vi "READ_SCOPETRACESENErgz analysis.vi"() -> ()   [LabVIEW 2011]
panel:
  out "results":dbl[][](array[numeric])
  out "Array":dbl[](array[numeric])
  in  "Export folder":bool
  in  "Export file":bool
  in  "Files":i32[](listbox)=[7]
  out "filenames":string[](array[string])=["TREX PXI slow_026.dat", "TREX PXI slow_027.dat", "TREX PXI slow_028.dat", "TREX PXI slow_029.dat", "TREX PXI slow_030.dat", "TREX PXI slow_031.dat", "TREX PXI slow_032.dat", "TREX PXI slow_033.dat", "TREX PXI slow_034.dat", "TREX PXI slow_035.dat", "TREX PXI slow_036.dat", "TREX PXI slow_037.dat", "TREX PXI slow_038.dat"]
  in  "pattern":string="*.dat"
  in  "Folder path":path=path "W:/USER/Thomas/temp"
  out "number of waveforms":i32=8
  out "ChannelNAmes":string[](array[string])=["0", "1", "2", "3", "4", "5", "6", "7"]
  in  "stop":bool
  in  "Channels":i32[](listbox)=[1]
  in  "file path (dialog if empty)":path=path "W:/USER/Thomas/temp/TREX PXI slow_033.dat"
  out "Waveform Graph":waveform(dbl)[](graph)=[{"t0"=timestamp(0 s since 1904-01-01), "dt"=1.6666666666666667e-08, "Y"=array[100000 elements], "attributes"=variant("Plot.Name"=variant(string "0"))}, {"t0"=timestamp(0 s since 1904-01-01), "dt"=1.6666666666666667e-08, "Y"=array[100000 elements], "attributes"=variant("Plot.Name"=variant(string "1"))}, {"t0"=timestamp(0 s since 1904-01-01), "dt"=1.6666666666666667e-08, "Y"=array[100000 elements], "attributes"=variant("Plot.Name"=variant(string "2"))}, {"t0"=timestamp(0 s since 1904-01-01), "dt"=1.6666666666666667e-08, "Y"=array[100000 elements], "attributes"=variant("Plot.Name"=variant(string "3"))}, {"t0"=timestamp(0 s since 1904-01-01), "dt"=1.6666666666666667e-08, "Y"=array[100000 elements], "attributes"=variant("Plot.Name"=variant(string "4"))}, {"t0"=timestamp(0 s since 1904-01-01), "dt"=1.6666666666666667e-08, "Y"=array[100000 elements], "attributes"=variant("Plot.Name"=variant(string "5"))}, {"t0"=timestamp(0 s since 1904-01-01), "dt"=1.6666666666666667e-08, "Y"=array[100000 elements], "attributes"=variant("Plot.Name"=variant(string "6"))}, {"t0"=timestamp(0 s since 1904-01-01), "dt"=1.6666666666666667e-08, "Y"=array[100000 elements], "attributes"=variant("Plot.Name"=variant(string "7"))}]
  out "error":string
  out "Slide":u8(slide)=1 scale=0.0..26.0
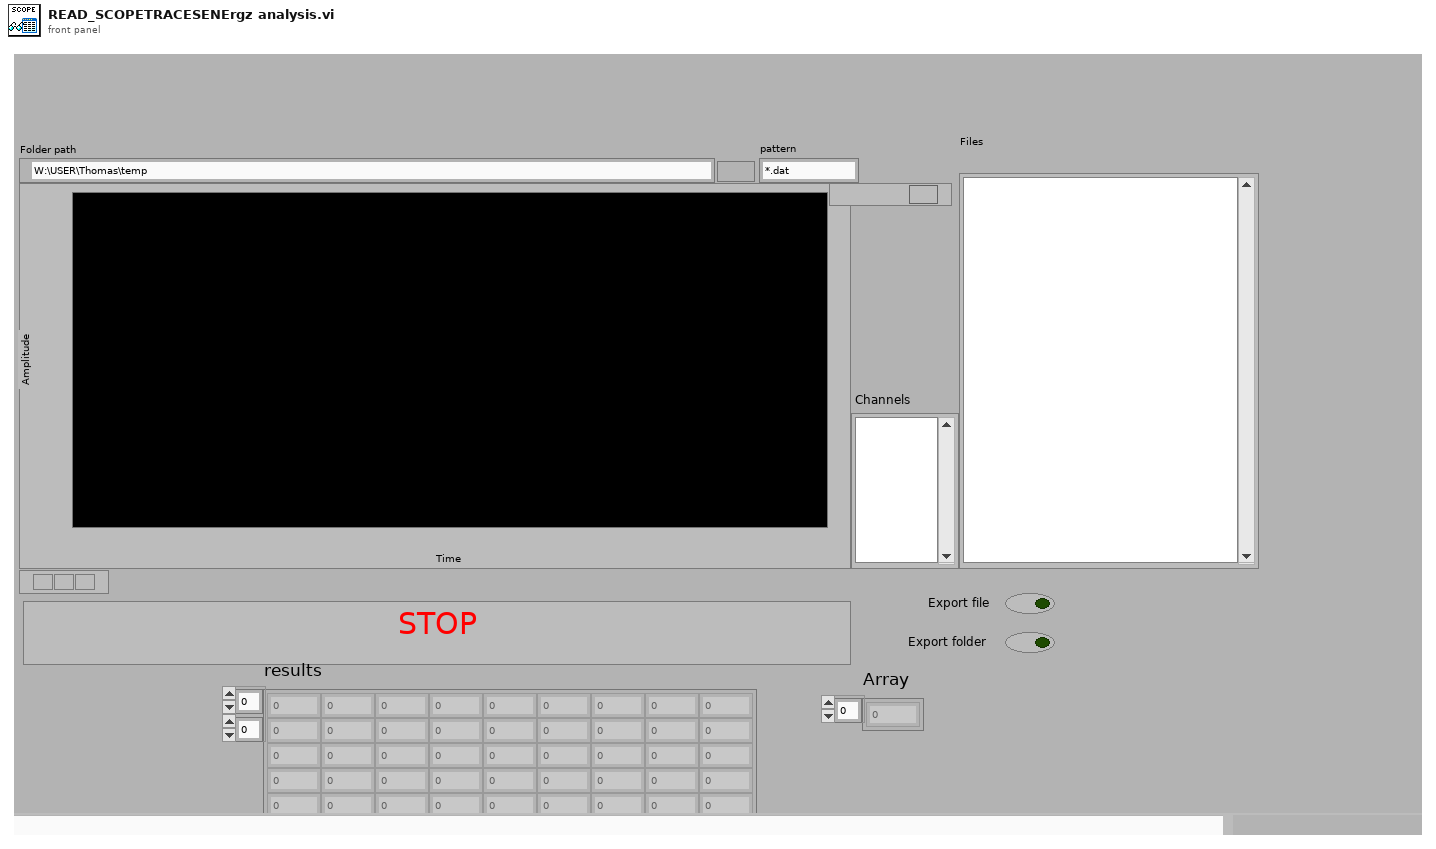
[diagram p1: front panel]
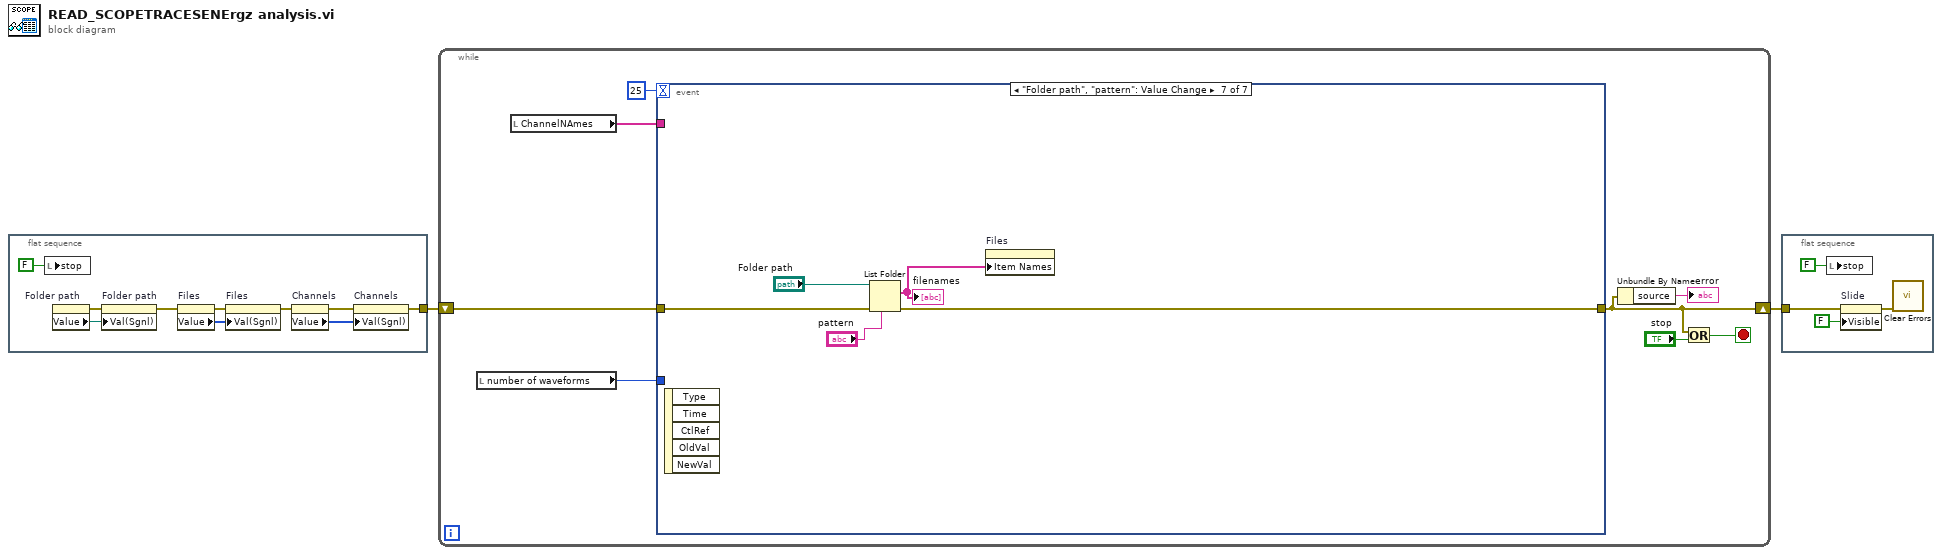
[diagram p0: block diagram]
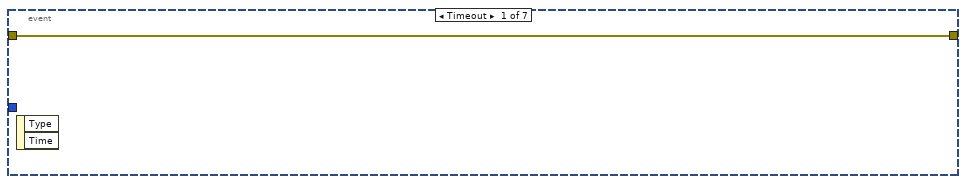
[diagram p2: hidden frame]
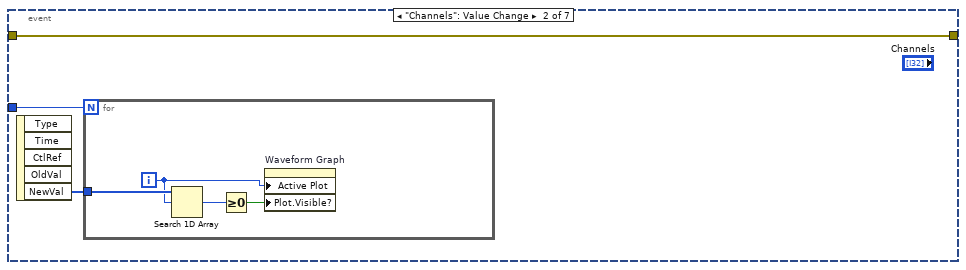
[diagram p3: hidden frame]
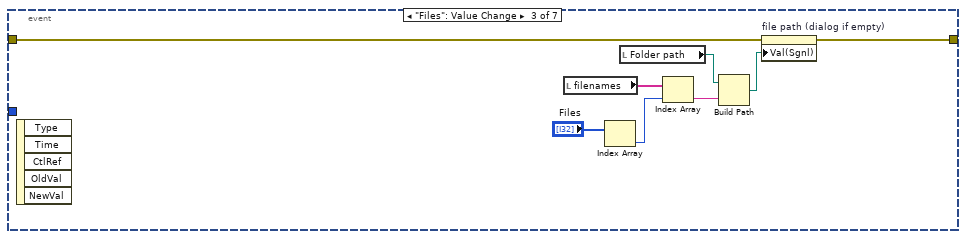
[diagram p4: hidden frame]
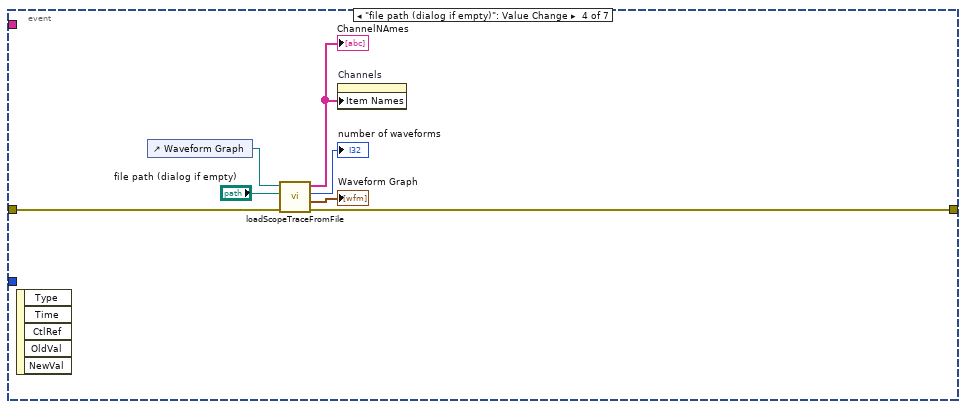
[diagram p5: hidden frame]
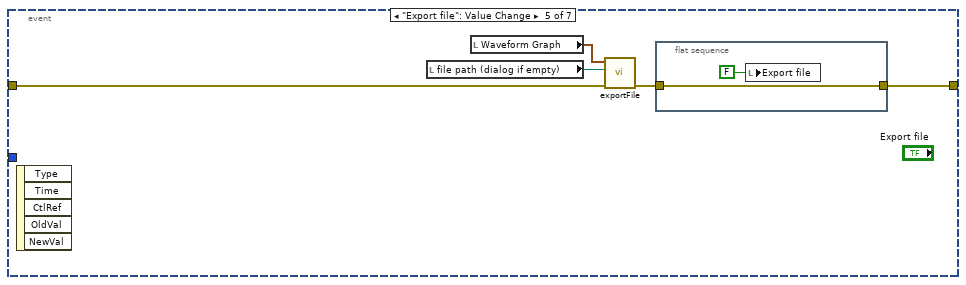
[diagram p6: hidden frame]
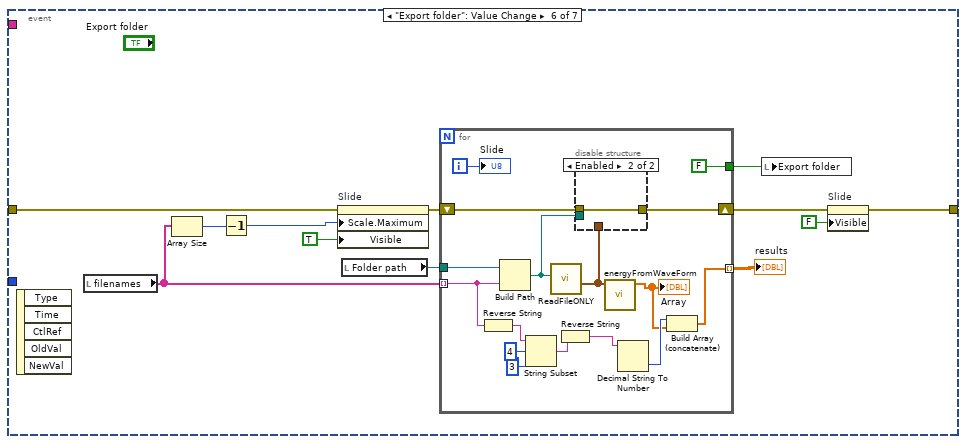
[diagram p7: hidden frame]
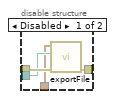
[diagram p8: hidden frame]
diagram:
  n1 = flat-sequence {
    tunnel: [w10] -> w2
    frame #0 {
      n2 = local write "stop"(FALSE ("stop")) -> ()
      n3 = property on="Folder path" class="Path"() -> (error out=w8:errorcluster, "Value"=w9:path)  [unwired: 2 in, 1 out]
      n4 = property on="Folder path" class="Path"(error in=w8, "Val(Sgnl)"=w9) -> (error out=w7:errorcluster)  [unwired: 1 in, 1 out]
      n5 = property on="Files" class="LstBox (strict)"(error in=w7) -> (error out=w6:errorcluster, "Value"=w4:i32[])  [unwired: 1 in, 1 out]
      n6 = property on="Files" class="LstBox (strict)"(error in=w6, "Val(Sgnl)"=w4) -> (error out=w5:errorcluster)  [unwired: 1 in, 1 out]
      n7 = property on="Channels" class="LstBox (strict)"(error in=w5) -> (error out=w11:errorcluster, "Value"=w12:i32[])  [unwired: 1 in, 1 out]
      n8 = property on="Channels" class="LstBox (strict)"(error in=w11, "Val(Sgnl)"=w12) -> (error out=w10:errorcluster)  [unwired: 1 in, 1 out]
    }
  }
  n9 = while {
    shift-right: [w15] -> w1
    shift-left: w2 -> [w17]
    stop <- w13 stop-if-true
    n10 = local read "number of waveforms"() -> (w18:i32)
    n11 = local read "ChannelNAmes"() -> (w19:string[])
    n12 = event shown="[6] \"Folder path \", \"pattern\": Value Change" {
      selector: _ -> [_ _ _ _ _ _ _]
      dyn-events: _ -> [_ _ _ _ _ _ _]
      timeout: 25 -> [_ _ _ _ _ _ _]
      tunnel: w19 -> [_ _ _ _ _ _ _]
      tunnel: w18 -> [_ w24 _ _ _ _ _]
      tunnel: [w21 w22 w29 w40 w44 w53 w84] -> w15
      tunnel: w17 -> [w21 w22 w30 w39 w45 w56 w85]
      event Timeout {
        n13 = event-data() -> ()  [unwired: 1 in, 2 out]
      }
      event "Channels": Value Change {
        n14 = event-data() -> ("NewVal"=w23:i32[])  [unwired: 1 in, 4 out]
        n15 = for {
          N: w24 -> [_]
          tunnel: w23 -> [w28]
          i -> [w27]
          n16 = Search 1D Array(1D array=w28, element=w27) -> (index of element=w26:i32)  [unwired: 1 in]
          n17 = Greater Or Equal To 0?(x=w26) -> (x >= 0?=w25:bool)
          n18 = property on="Waveform Graph" class="WFGraph (strict)"("Active Plot"=w27, "Plot.Visible?"=w25) -> ()  [unwired: 2 in, 2 out]
        }
      }
      event "Files": Value Change {
        n19 = event-data() -> ()  [unwired: 1 in, 5 out]
        n20 = local read "filenames"() -> (w36:string[])
        n21 = Index Array(array="Files") -> (element=w34:i32)  [unwired: 1 in]
        n22 = local read "Folder path"() -> (w33:path)
        n23 = Index Array(array=w36, index=w34) -> (element=w32:string)
        n24 = Build Path(base path=w33, name or relative path=w32) -> (appended path=w31:path)
        n25 = property on="file path (dialog if empty)" class="Path"(error in=w30, "Val(Sgnl)"=w31) -> (error out=w29:errorcluster)  [unwired: 1 in, 1 out]
      }
      event "file path (dialog if empty)": Value Change {
        n26 = event-data() -> ()  [unwired: 1 in, 5 out]
        n27 = control-ref of="Waveform Graph"() -> (w43:refnum<vi>)
        n28 = call "loadScopeTraceFromFile.vi"("error in (no error)"=w39, "file path (dialog if empty)"="file path (dialog if empty)", "WaveformGraph in"=w43) -> ("error out"=w40:errorcluster, "Array 2"=→"Waveform Graph":waveform(dbl)[], "number of waveforms"=→"number of waveforms":i32, "Array"=w38:string[])  [unwired: 5 in]
        "ChannelNAmes" <- w38
        n29 = property on="Channels" class="LstBox (strict)"("Item Names"=w38) -> ()  [unwired: 2 in, 2 out]
      }
      event "Export file": Value Change {
        n30 = event-data() -> ()  [unwired: 1 in, 5 out]
        n31 = local read "file path (dialog if empty)"() -> (w47:path)
        n32 = local read "Waveform Graph"() -> (w48:waveform(dbl)[])
        n33 = call "exportFile.vi"("error in"=w45, "file path (dialog if empty)"=w47, "Waveform Graph"=w48) -> ("error out"=w46:errorcluster)  [unwired: 8 in]
        n34 = flat-sequence {
          tunnel: w46 -> [w49]
          tunnel: [w49] -> w44
          frame #0 {
            n35 = local write "Export file"(FALSE) -> ()
          }
        }
      }
      event "Export folder": Value Change {
        n36 = event-data() -> ()  [unwired: 1 in, 5 out]
        n37 = local read "filenames"() -> (w60:string[])
        n38 = Array Size(array=w60) -> (size(s)=w59:i32)
        n39 = Decrement(x=w59) -> (x-1=w58:i32)
        n40 = property on="Slide" class="Slide (strict)"(error in=w56, "Scale.Maximum"=w58, "Visible"=TRUE) -> (error out=w55:errorcluster)  [unwired: 1 in, 1 out]
        n41 = local read "Folder path"() -> (w62:path)
        n42 = for {
          tunnel: w60 -> [w71] mode=indexing
          tunnel: w62 -> [w78]
          tunnel: [FALSE] -> w61
          shift-right: [w75] -> w54
          shift-left: w55 -> [w76]
          tunnel: [w63] -> w51 mode=indexing
          i -> [w73]
          n43 = Reverse String(1:w71) -> (0:w70:string)
          n44 = Build Path(base path=w78, name or relative path=w71) -> (appended path=w74:path)
          n45 = String Subset(string=w70, offset (0)=4, length (rest)=3 ("length (rest)")) -> (substring=w67:string)
          n46 = call "ReadFileONLY.vi"("file path (dialog if empty)"=w74) -> ("Array 2"=w72:waveform(dbl)[])  [unwired: 7 in, 3 out]
          n47 = Reverse String(1:w67) -> (0:w66:string)
          n48 = disable-structure shown="Enabled" {
            disable-tunnel: w76 -> [w82 w83]
            disable-tunnel: [w81 w83] -> w75
            disable-tunnel: w74 -> [w80 _]
            disable-tunnel: w72 -> [w79 _]
            frame Disabled {
              n49 = call "exportFile.vi"("error in"=w82, "file path (dialog if empty)"=w80, "Waveform Graph"=w79) -> ("error out"=w81:errorcluster)  [unwired: 8 in]
            }
            frame Enabled {
            }
          }
          n50 = call "energyFromWaveForm.vi"("Array in"=w72) -> ("results"=w64:dbl[])  [unwired: 10 in]
          "Array" <- w64
          n51 = Decimal String To Number(string=w66) -> (number=w65:i32)  [unwired: 2 in, 1 out]
          n52 = Build Array (concatenate)(w65, w64) -> (w63:dbl[])
          "Slide" <- w73
        }
        "results" <- w51
        n53 = local write "Export folder"(w61) -> ()
        n54 = property on="Slide" class="Slide (strict)"(error in=w54, "Visible"=FALSE) -> (error out=w53:errorcluster)  [unwired: 1 in, 1 out]
      }
      event "Folder path", "pattern": Value Change {
        n55 = event-data() -> ()  [unwired: 1 in, 5 out]
        n56 = List Folder(path="Folder path", pattern="pattern", error in=w85) -> (filenames=w88:string[], error out=w84:errorcluster)  [unwired: 1 in, 2 out]
        "filenames" <- w88
        n57 = property on="Files" class="LstBox (strict)"("Item Names"=w88) -> ()  [unwired: 2 in, 2 out]
      }
    }
    n58 = Unbundle By Name(w15) -> ("source"=→"error":string)
    n59 = Or(x=w15, y="stop") -> (x .or. y?=w13:bool)
  }
  n60 = flat-sequence {
    tunnel: w1 -> [w92]
    frame #0 {
      n61 = local write "stop"(FALSE ("stop")) -> ()
      n62 = property on="Slide" class="Slide (strict)"(error in=w92, "Visible"=FALSE) -> (error out=w89:errorcluster)  [unwired: 1 in, 1 out]
      n63 = call <vilib>:"Clear Errors.vi"("error in (no error)"=w89) -> ()  [unwired: 6 in, 1 out]
    }
  }
